vi "VI Path Test App.vi"() -> ()   [LabVIEW 2011]
uses:
  LVH-Build-Tools.lvlib
panel:
  out "VI Path":path
  in  "Error In":errorcluster
  out "Numeric Control":i32
  in  "Stop Button":bool
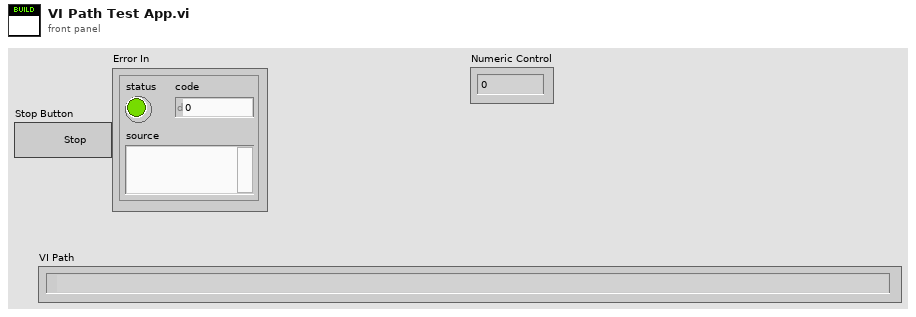
[diagram p1: front panel]
types:
  T1 = typedef "LVH-Toolbox.lvlib/LVH-Build-Tools.lvlib/Sync Source Configuration.ctl" = cluster{"Installed Projects":T2[], "Project Source Root Dir":path, "All Config Files":path[], "Selected Project Config":path, "All LabVIEW Dirs":path[], "Selected LabVIEW Dir":path, "Backup Dir":path}
  T2 = typedef "LVH-Toolbox.lvlib/LVH-Build-Tools.lvlib/Installed Project.ctl" = cluster{"Project Name":string, "LV Versions":T3[], "Project Config Path":path}
  T3 = typedef "LVH-Toolbox.lvlib/LVH-SystemTools.lvlib/Installed LabVIEW Version.ctl" = cluster{"Version":string, "Path":path}
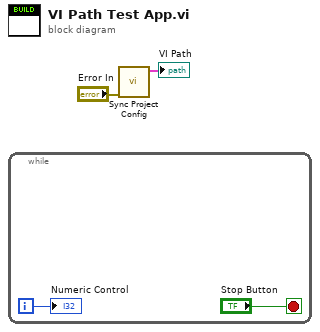
[diagram p0: block diagram]
diagram:
  n1 = while {
    i -> [w3]
    stop <- "Stop Button" stop-if-true
    "Numeric Control" <- w3
  }
  n2 = call "Sync Project Config.vi"("Error In"="Error In") -> ("Sync Source Config"=→"VI Path":T1)  [unwired: 9 in, 1 out]
